vi "PDF Konfig EPA-Dichtheitstest.vi"(8 "error in (no error)":errorcluster caption="Fehler (Eingang, kein Fehler)", 10 "Failed":bool, 11 "seconds since 1Jan1904":timestamp) -> (0 "error out":errorcluster caption="Fehler (Ausgang)", 3 "PDF Pfad":path)   [LabVIEW 2020, in "EPA 1065.lvlib" / "Dichtheitstest 1065-345.lvlib"]
uses:
  Dichtheitstest 1065-345.lvlib
  Sprachverwaltung/FGV Aktion Tabelle zerlegen.ctl
  Linearisierung V2/Protokoll/Protokoll.lvlib
  Sprachverwaltung/Sprachverwaltung.lvlib
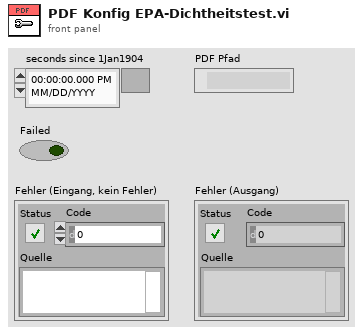
[diagram p1: front panel]
types:
  T1 = typedef "Sprachverwaltung.lvlib/FGV Aktion Tabelle zerlegen.ctl" = enum16{"laden", "vereinzeln", "speichern"}
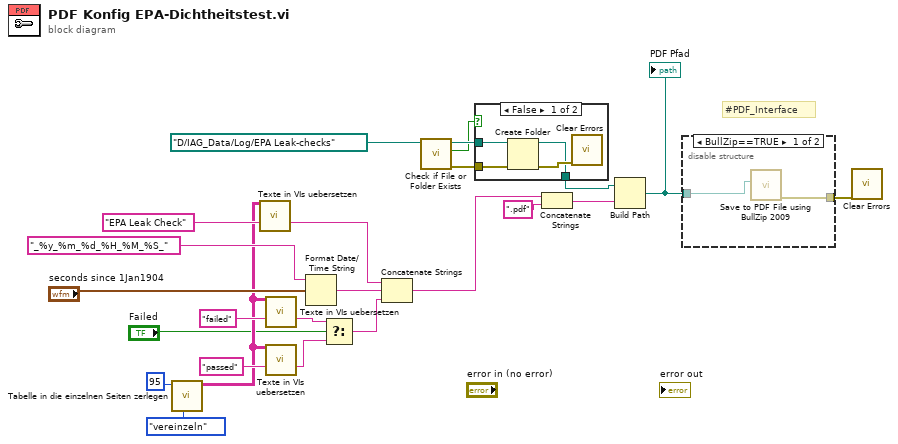
[diagram p0: block diagram]
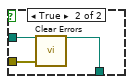
[diagram p2: hidden frame]
diagram:
  # "#PDF_Interface"
  n1 = call "Tabelle in die einzelnen Seiten zerlegen.vi"("Aktion"=FGV_Aktion_Tabelle_zerlegen."vereinzeln", "Index (Seite)"=95) -> ("Sprachliste"=w2:string[][])  [unwired: 7 in, 2 out]
  n2 = call "Texte in VIs uebersetzen.vi"("Sprachliste"=w2, "String zum Übersetzen"="EPA Leak Check" ("String")) -> ("String zum Übersetzen"=w8:string)  [unwired: 9 in, 4 out]
  n3 = call "Texte in VIs uebersetzen.vi"("Sprachliste"=w2, "String zum Übersetzen"="failed" ("String")) -> ("String zum Übersetzen"=w4:string)  [unwired: 9 in, 4 out]
  n4 = call "Texte in VIs uebersetzen.vi"("Sprachliste"=w2, "String zum Übersetzen"="passed" ("String")) -> ("String zum Übersetzen"=w3:string)  [unwired: 9 in, 4 out]
  n5 = Format Date/Time String(time format string (%c)="_%y_%m_%d_%H_%M_%S_" ("Zeitformatierungs-String (%c)"), seconds (now)="seconds since 1Jan1904") -> (date/time string=w15:string)  [unwired: 1 in]
  n6 = Select(t=w4, s="Failed", f=w3) -> (s? t:f=w7:string)
  n7 = Concatenate Strings(w8, w15, w7) -> (w17:string)
  n8 = call <vilib>:"Check if File or Folder Exists.vi"("path"=path "D:/IAG_Data/Log/EPA Leak-checks" ("Pfad:")) -> ("error out"=w24:errorcluster, "file or folder exists?"=w21:bool, "dup path"=w22:path)  [unwired: 8 in]
  n9 = case shown="False" w21 {
    tunnel: w22 -> [w28 w30]
    tunnel: [w26 w30] -> w23
    tunnel: w24 -> [w25 w29]
    frame False {
      n10 = Create Folder(path (use dialog)=w28, error in=w25) -> (created path=w26:path, error out=w27:errorcluster)  [unwired: 1 in, 1 out]
      n11 = call <vilib>:"Clear Errors.vi"("error in (no error)"=w27) -> ()  [unwired: 5 in, 2 out]
    }
    frame True {
      n12 = call <vilib>:"Clear Errors.vi"("error in (no error)"=w29) -> ()  [unwired: 5 in, 2 out]
    }
  }
  n13 = Concatenate Strings(w17, ".pdf" ("String")) -> (w12:string)
  n14 = Build Path(base path=w23, name or relative path=w12) -> (appended path=w18:path)
  "PDF Pfad" <- w18
  n15 = disable-structure shown="BullZip==TRUE" {
    disable-tunnel: [w32 _] -> w19
    disable-tunnel: w18 -> [w31 _]
    frame condition #0 {
      n16 = call "Save to PDF File using BullZip 2009.vi"("Save PDF File Path"=w31) -> ("error out"=w32:errorcluster)  [unwired: 10 in]
    }
    frame condition #1 (active) {
    }
  }
  n17 = call <vilib>:"Clear Errors.vi"("error in (no error)"=w19) -> ()  [unwired: 5 in, 2 out]
